vi "error decide.vi"(10 "date/time string":string, 11 "date/time string 2":string) -> (3 "String":string)   [LabVIEW 2018]
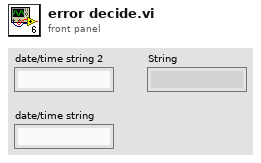
[diagram p1: front panel]
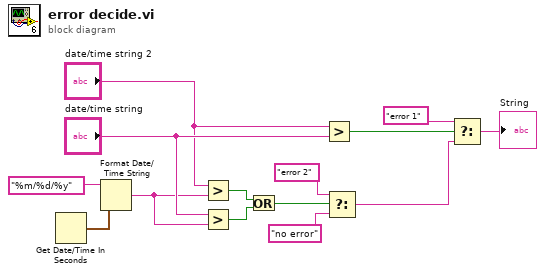
[diagram p0: block diagram]
diagram:
  n1 = Get Date/Time In Seconds() -> (seconds since 1Jan1904=w1:timestamp)
  n2 = Format Date/Time String(time format string (%c)="%m/%d/%y", seconds (now)=w1) -> (date/time string=w9:string)  [unwired: 1 in]
  n3 = Greater?(x="date/time string 2", y=w9) -> (0:w3:bool)
  n4 = Greater?(x="date/time string", y=w9) -> (0:w4:bool)
  n5 = Or(x=w3, y=w4) -> (x .or. y?=w5:bool)
  n6 = Greater?(x="date/time string 2", y="date/time string") -> (0:w14:bool)
  n7 = Select(t="error 2", s=w5, f="no error") -> (s? t:f=w11:string)
  n8 = Select(t="error 1", s=w14, f=w11) -> (s? t:f=→"String":string)
